vi "main 5th.vi"() -> ()   [LabVIEW 2013]
panel:
  out "From OD fit?":bool
  in  "Current file num":i32
  in  "Fitting Results Save Path":string[](array[string])
  in  "Initial guess values":dbl[](array[numeric])
  out "Latest image data":dbl[][](array[numeric])
  in  "Fitting Type":u16(ring)
  in  "Force Guess?":bool
  out "best fit parameters":dbl[](array[numeric])
  in  "Reset process index":bool
  out "ROI Height":u32
  out "ROI Width":u32
  out "OD image":dbl[][](graph)
  out "Process Index":i32
  out "External Trigger":bool
  out "XY图":cluster{i32[], dbl[]}[](graph)
  in  "OD fit":bool
  in  "OD num":i32
  out "Fit Done":bool
  in  "Exit":bool
  out "XY图 2":cluster{i32[], dbl[]}[](graph)
  in  "Auto Split":bool
  in  "Fit":bool
  in  "Open File":bool
  in  "Auto Fit":bool
  in  "Stop":bool
  in  "Aquire":bool
  in  "Fitting Config":bool
  in  "Camera Config":bool
  in  "Initialize":bool
  in  "Live Image Display":refnum<k7>(container)
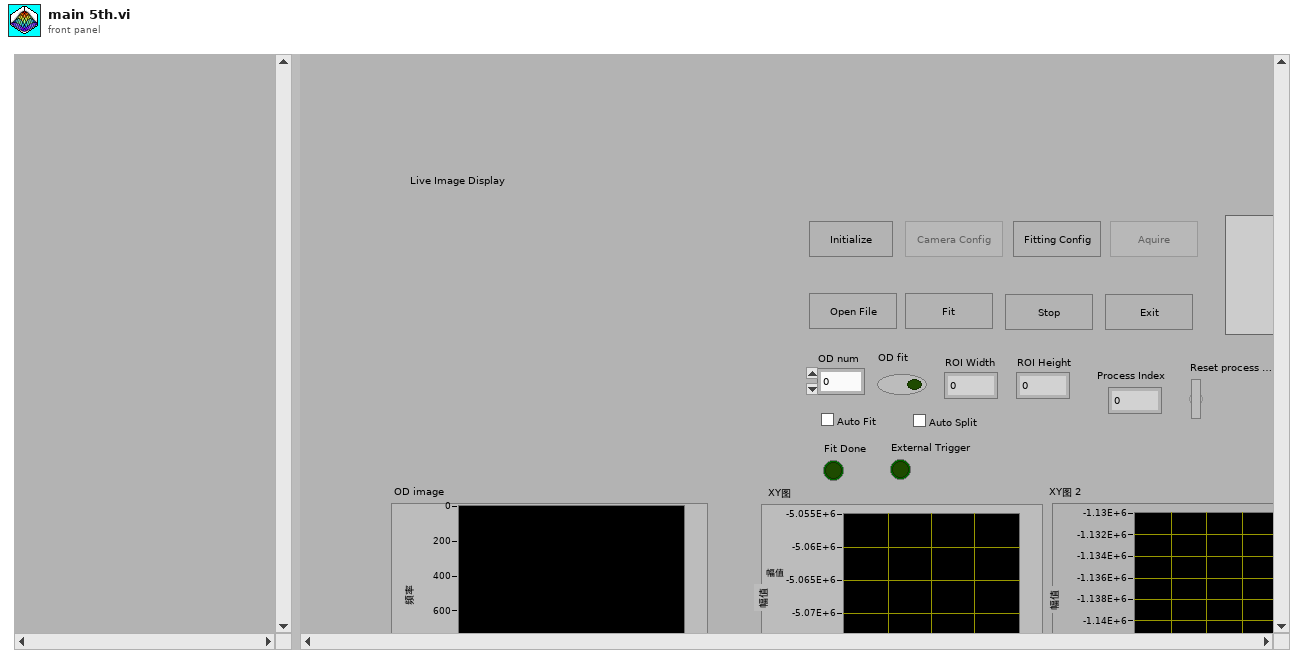
[diagram p1: front panel]
types:
  T1 = enum8{"Enabled", "Disabled", "Disabled and Grayed Out"}
  T2 = typedef "Image Type" = u32
  T3 = typedef "IMAQ Image.ctl" = refnum<image>
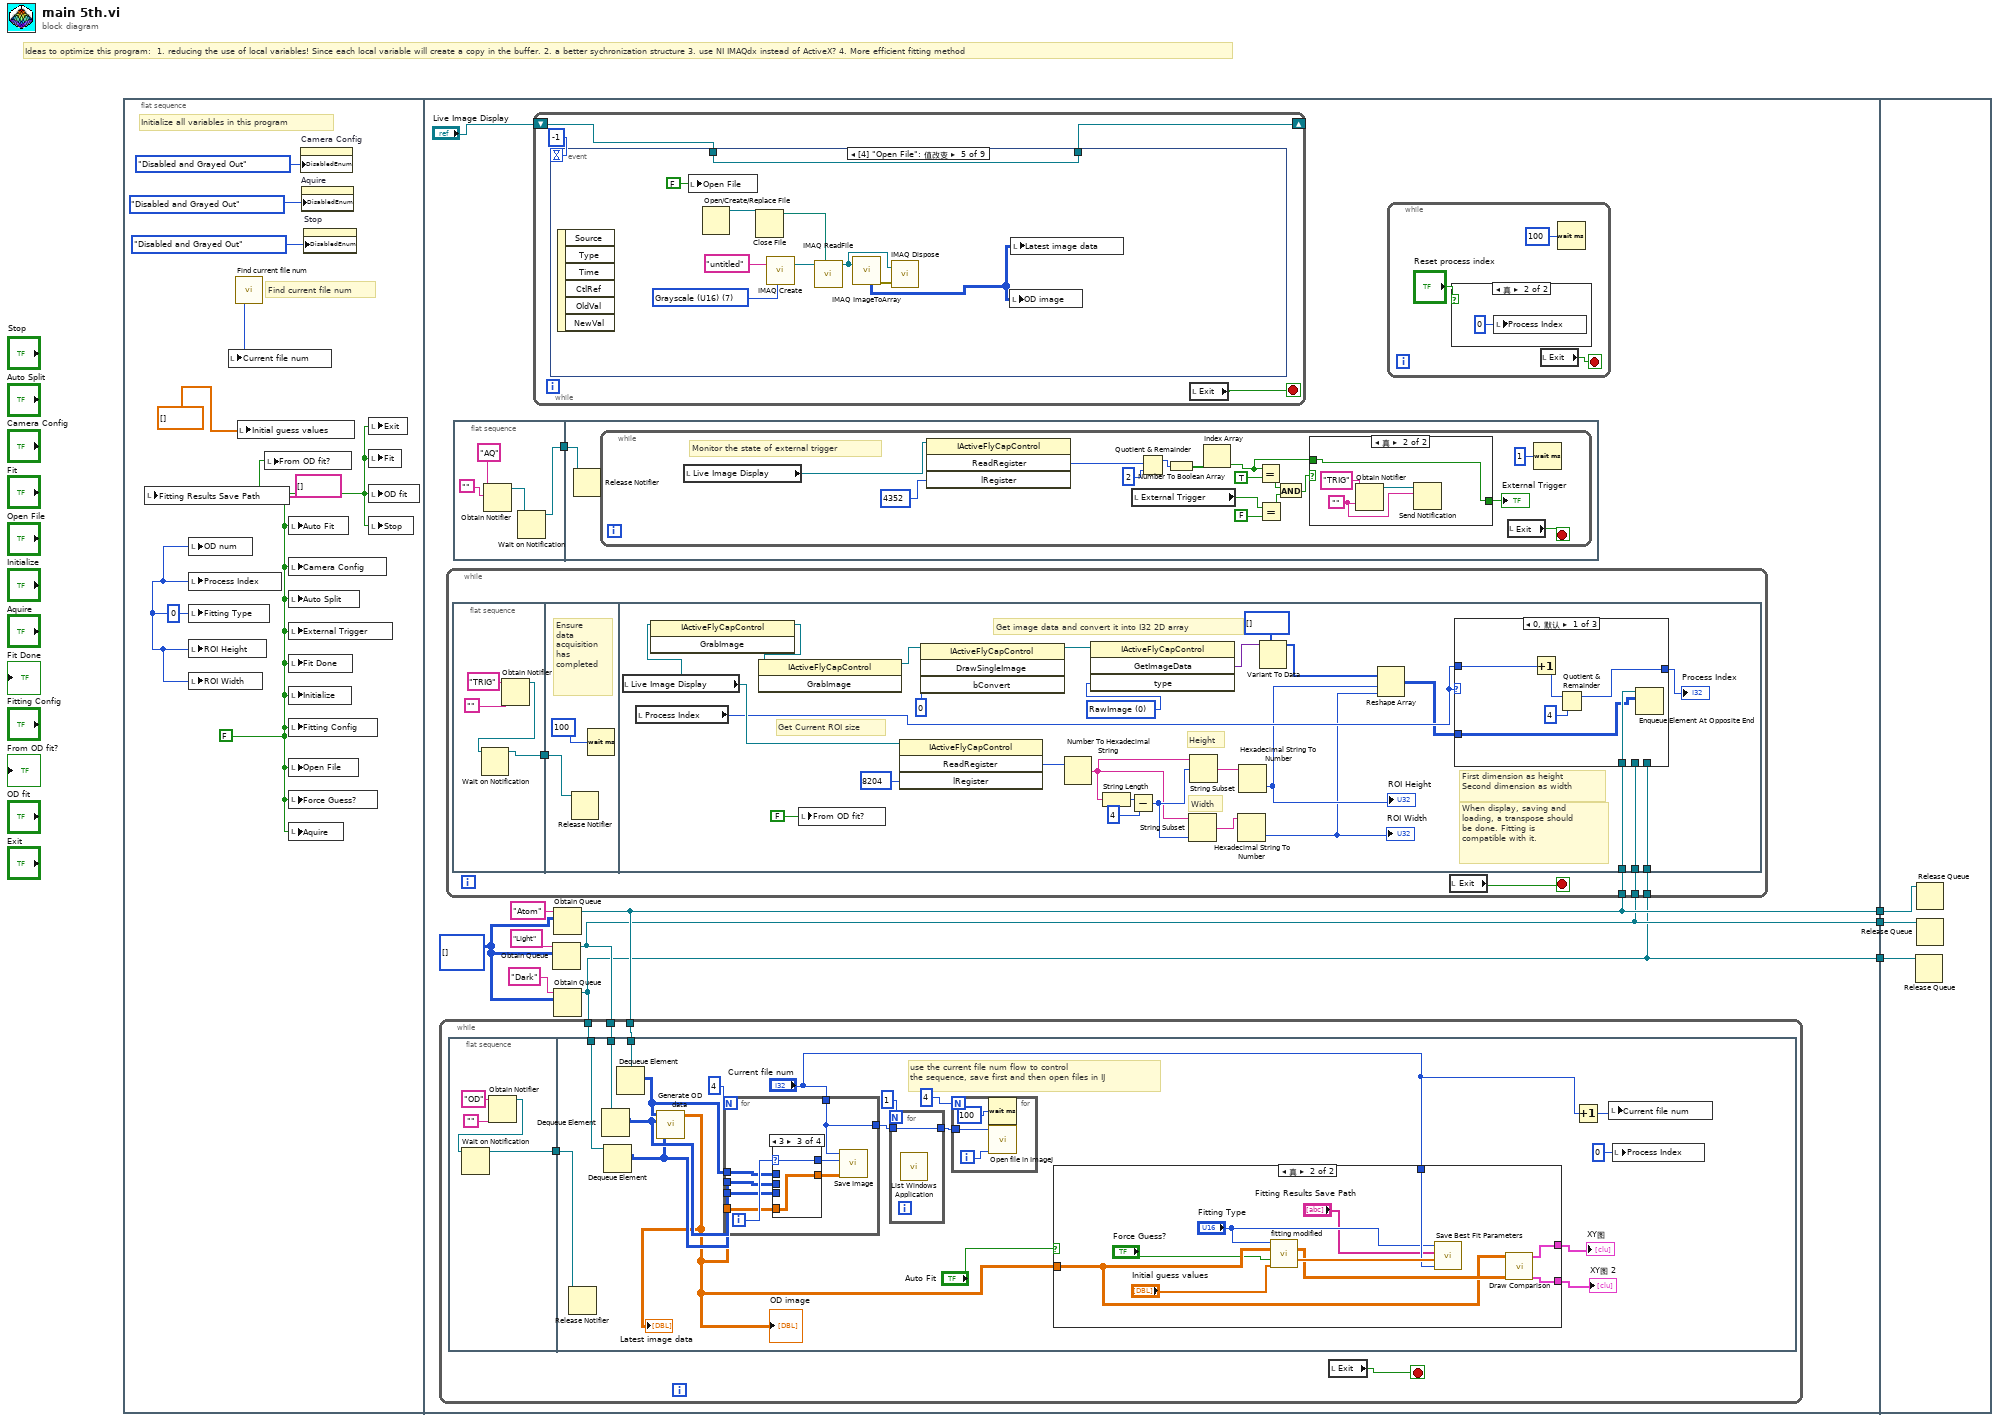
[diagram p0: block diagram]
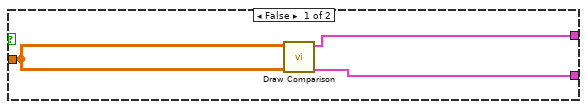
[diagram p3: hidden frame]
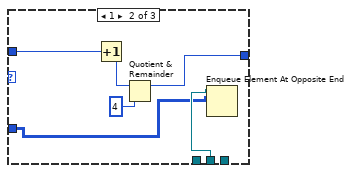
[diagram p8: hidden frame]
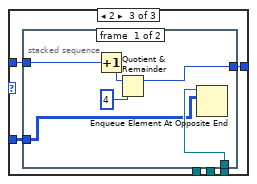
[diagram p9: hidden frame]
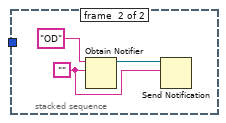
[diagram p10: hidden frame]
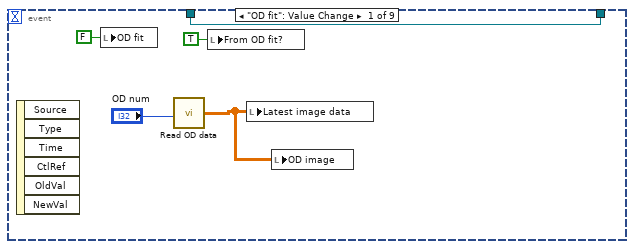
[diagram p11: hidden frame]
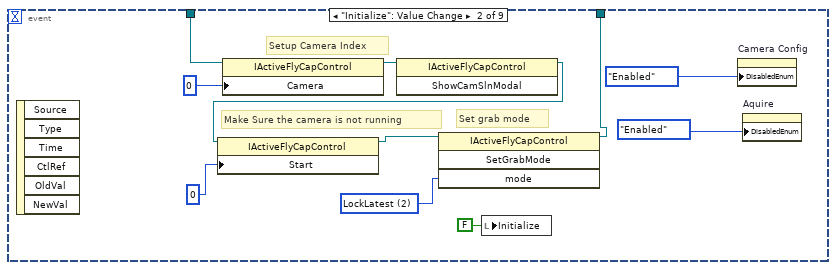
[diagram p12: hidden frame]
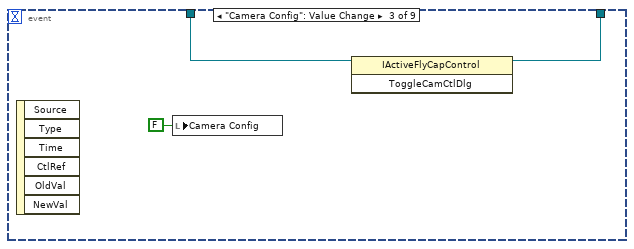
[diagram p13: hidden frame]
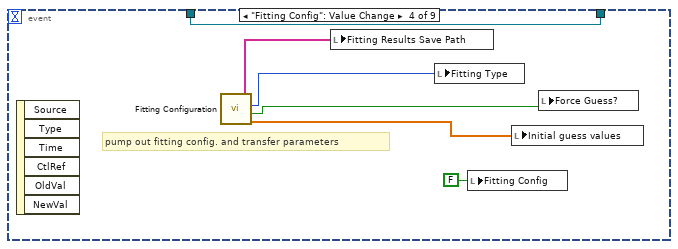
[diagram p14: hidden frame]
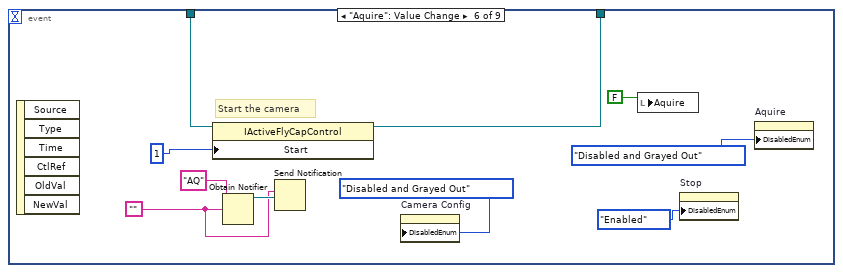
[diagram p15: hidden frame]
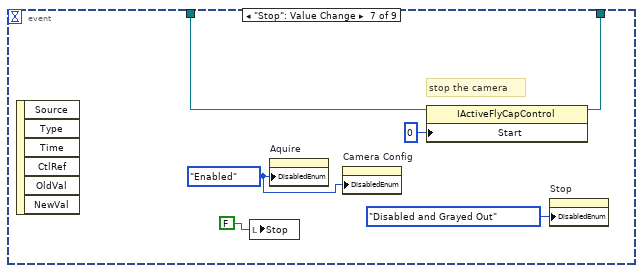
[diagram p16: hidden frame]
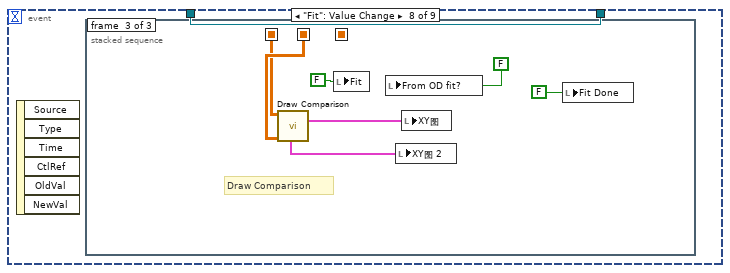
[diagram p17: hidden frame]
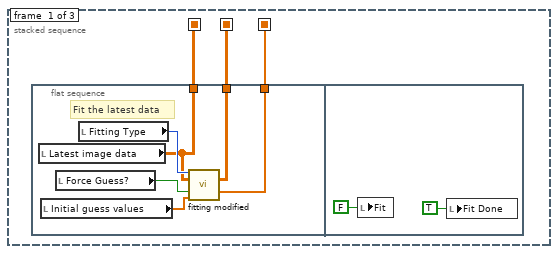
[diagram p18: hidden frame]
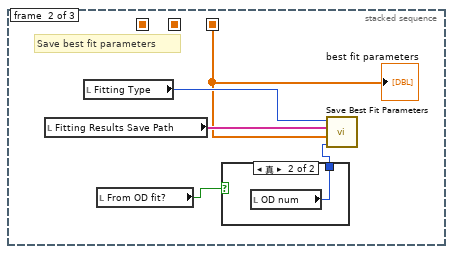
[diagram p19: hidden frame]
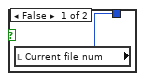
[diagram p20: hidden frame]
diagram:
  # "Ideas to optimize this program:  1. reducing the use of local variables! Since each local variable will create a copy in the buffer. 2. a better sychronization structure 3. use NI IMAQdx instead of ActiveX? 4. More efficient fitting method"
  n1 = flat-sequence {
    tunnel: [w15] -> w3
    tunnel: [w14] -> w2
    tunnel: [w13] -> w1
    tunnel: w3 -> [w258]
    tunnel: w2 -> [w257]
    tunnel: w1 -> [w256]
    frame #0 {
      w7 = 0 ("OD num")
      w5 = FALSE ("Aquire")
      # "Find current file num"
      # "Initialize all variables in this program"
      n2 = local write "Fitting Results Save Path"(string[] [] ("Fitting Results Save Path")) -> ()
      n3 = local write "OD num"(w7) -> ()
      n4 = local write "Process Index"(w7) -> ()
      n5 = local write "Fitting Type"(w7) -> ()
      n6 = local write "ROI Height"(w7) -> ()
      n7 = local write "ROI Width"(w7) -> ()
      n8 = call "Find current file num.vi"() -> ("Current File Num"=w4:u16)  [unwired: 2 in]
      n9 = local write "Current file num"(w4) -> ()
      n10 = local write "Initial guess values"(dbl[] [] ("Best fit parameters")) -> ()
      n11 = local write "From OD fit?"(w5) -> ()
      n12 = local write "Auto Fit"(w5) -> ()
      n13 = local write "Camera Config"(w5) -> ()
      n14 = local write "Auto Split"(w5) -> ()
      n15 = local write "External Trigger"(w5) -> ()
      n16 = local write "Fit Done"(w5) -> ()
      n17 = local write "Initialize"(w5) -> ()
      n18 = local write "Fitting Config"(w5) -> ()
      n19 = local write "Open File"(w5) -> ()
      n20 = local write "Force Guess?"(w5) -> ()
      n21 = local write "Aquire"(w5) -> ()
      n22 = property on="Camera Config" class="Bool (严格)"("DisabledEnum"=T1."Disabled and Grayed Out" ("禁用")) -> ()  [unwired: 2 in, 2 out]
      n23 = property on="Aquire" class="Bool (严格)"("DisabledEnum"=T1."Disabled and Grayed Out" ("禁用")) -> ()  [unwired: 2 in, 2 out]
      n24 = property on="Stop" class="Bool (严格)"("DisabledEnum"=T1."Disabled and Grayed Out" ("禁用")) -> ()  [unwired: 2 in, 2 out]
      n25 = local write "Exit"(w5) -> ()
      n26 = local write "Fit"(w5) -> ()
      n27 = local write "OD fit"(w5) -> ()
      n28 = local write "Stop"(w5) -> ()
    }
    frame #1 {
      w16 = i32[][] [] ("输出数组")
      n29 = flat-sequence {
        tunnel: [w86] -> w20
        tunnel: w20 -> [w90]
        frame #0 {
          n30 = Obtain Notifier(name (unnamed)="AQ" ("名称（未命名）"), notification data type="") -> (notifier out=w88:refnum<notifier>)  [unwired: 2 in, 2 out]
          n31 = Wait on Notification(notifier=w88) -> (notifier out=w86:refnum<notifier>)  [unwired: 3 in, 3 out]
        }
        frame #1 {
          n32 = Release Notifier(notifier=w90) -> ()  [unwired: 2 in, 3 out]
          n33 = while {
            stop <- w106 stop-if-true
            # "Monitor the state of external trigger"
            n34 = local read "Live Image Display"() -> (w105:refnum<k7>)
            n35 = invoke class="IActiveFlyCapControl" method="ReadRegister"(reference=w105, "lRegister"=u32 4352) -> ("ReadRegister"=w103:u32)  [unwired: 2 in, 3 out]
            n36 = local read "External Trigger"() -> (w98:bool)
            n37 = Quotient & Remainder(x=w103, y=u32 2) -> (x-y*floor(x/y)=w101:u32)  [unwired: 1 out]
            n38 = Number To Boolean Array(number=w101) -> (Boolean array=w100:bool[])
            n39 = Index Array(array=w100) -> (element=w93:bool)  [unwired: 1 in]
            n40 = Equal?(x=w93, y=TRUE) -> (x = y?=w95:bool)
            n41 = Equal?(x=w98, y=FALSE) -> (x = y?=w96:bool)
            n42 = And(x=w95, y=w96) -> (x .and. y?=w94:bool)
            n43 = case shown="真" w94 {
              tunnel: w93 -> [w107 w108]
              tunnel: [w107 w108] -> w91
              frame False {
              }
              frame True {
                w109 = ""
                n44 = Obtain Notifier(name (unnamed)="TRIG" ("名称（未命名）"), notification data type=w109) -> (notifier out=w110:refnum<notifier>)  [unwired: 2 in, 2 out]
                n45 = Send Notification(notification=w109, notifier=w110) -> ()  [unwired: 1 in, 2 out]
              }
            }
            "External Trigger" <- w91
            n46 = local read "Exit"() -> (w106:bool)
            n47 = Wait (ms)(milliseconds to wait=u32 1 ("等待时间（毫秒）")) -> ()  [unwired: 1 out]
          }
        }
      }
      n48 = while {
        shift-right: [w174] -> _
        shift-left: "Live Image Display" -> [w175]
        stop <- w177 stop-if-true
        n49 = event shown="[4] \"Open File\": 值改变" {
          selector: _ -> [_ _ _ _ _ _ _ _ _]
          dyn-events: _ -> [_ _ _ _ _ _ _ _ _]
          timeout: -1 -> [_ _ _ _ _ _ _ _ _]
          tunnel: w175 -> [w178 w187 w195 w197 w211 w214 w225 w229 w255]
          tunnel: [w178 w183 w194 w197 w211 w213 w224 w229 w255] -> w174
          event "OD fit": Value Change {
            n50 = event-data() -> ()  [unwired: 1 in, 6 out]
            n51 = local write "OD fit"(FALSE ("OD fit")) -> ()
            n52 = call "Read OD data.vi"("OD num"="OD num") -> ("OD data"=w180:dbl[][])  [unwired: 4 in]
            n53 = local write "From OD fit?"(TRUE ("From OD fit?")) -> ()
            n54 = local write "Latest image data"(w180) -> ()
            n55 = local write "OD image"(w180) -> ()
          }
          event "Initialize": Value Change {
            w191 = 2 items=["FreeRunning", "LockNext", "LockLatest"] ("mode")
            # "Setup Camera Index"
            # "Set grab mode"
            # "Make Sure the camera is not running"
            n56 = event-data() -> ()  [unwired: 1 in, 6 out]
            n57 = property class="IActiveFlyCapControl"(reference=w187, "Camera"=0 ("Start")) -> (reference out=w190:refnum<k7>)  [unwired: 1 in, 1 out]
            n58 = invoke class="IActiveFlyCapControl" method="ShowCamSlnModal"(reference=w190) -> (reference out=w186:refnum<k7>)  [unwired: 2 in, 2 out]
            n59 = property class="IActiveFlyCapControl"(reference=w186, "Start"=0 ("Camera")) -> (reference out=w185:refnum<k7>)  [unwired: 1 in, 1 out]
            n60 = invoke class="IActiveFlyCapControl" method="SetGrabMode"(reference=w185, "mode"=w191) -> (reference out=w183:refnum<k7>)  [unwired: 2 in, 3 out]
            n61 = local write "Initialize"(FALSE ("Initialize")) -> ()
            n62 = property on="Camera Config" class="Bool (严格)"("DisabledEnum"=T1."Enabled" ("禁用")) -> ()  [unwired: 2 in, 2 out]
            n63 = property on="Aquire" class="Bool (严格)"("DisabledEnum"=T1."Enabled" ("禁用")) -> ()  [unwired: 2 in, 2 out]
          }
          event "Camera Config": Value Change {
            n64 = event-data() -> ()  [unwired: 1 in, 6 out]
            n65 = local write "Camera Config"(FALSE ("Camera Config")) -> ()
            n66 = invoke class="IActiveFlyCapControl" method="ToggleCamCtlDlg"(reference=w195) -> (reference out=w194:refnum<k7>)  [unwired: 2 in, 2 out]
          }
          event "Fitting Config": Value Change {
            # "pump out fitting config. and transfer parameters"
            n67 = event-data() -> ()  [unwired: 1 in, 6 out]
            n68 = call "Fitting Configuration.vi"() -> ("intial guess"=w198:dbl[], "Force Guess？"=w199:bool, "Fitting Type"=w201:u16, "Fitting Results Save Path"=w200:string[])  [unwired: 5 in]
            n69 = local write "Fitting Results Save Path"(w200) -> ()
            n70 = local write "Fitting Type"(w201) -> ()
            n71 = local write "Fitting Config"(FALSE ("Fitting Config")) -> ()
            n72 = local write "Initial guess values"(w198) -> ()
            n73 = local write "Force Guess?"(w199) -> ()
          }
          event "Open File": Value Change {
            w210 = T2 7 items=["Grayscale (U8)", "Grayscale (I16)", "Grayscale (SGL)", "Complex (CSG)", "RGB (U32)", "HSL (U32)", "RGB (U64)", "Grayscale (U16)"] ("Image Type")
            n74 = event-data() -> ()  [unwired: 1 in, 6 out]
            n75 = local write "Open File"(FALSE ("Open File")) -> ()
            n76 = Open/Create/Replace File() -> (refnum out=w204:refnum<file>)  [unwired: 6 in, 2 out]
            n77 = Close File(refnum=w204) -> (path=w203:path)  [unwired: 1 in, 1 out]
            n78 = call "IMAQ Create"("Image Name"="untitled", "Image Type"=w210) -> ("New Image"=w209:T3)  [unwired: 3 in, 1 out]
            n79 = call "IMAQ ReadFile"("File Path"=w203, "Image"=w209) -> ("Image Out"=w208:T3)  [unwired: 5 in, 4 out]
            n80 = call "IMAQ ImageToArray"("Image"=w208) -> ("Image Pixels (U16)"=w205:u16[][], "error out"=w207:errorcluster)  [unwired: 3 in, 3 out]
            n81 = call "IMAQ Dispose"("Image"=w208, "error in (no error)"=w207) -> ()  [unwired: 4 in, 1 out]
            n82 = local write "OD image"(w205) -> ()
            n83 = local write "Latest image data"(w205) -> ()
          }
          event "Aquire": Value Change {
            w216 = ""
            # "Start the camera"
            n84 = event-data() -> ()  [unwired: 1 in, 6 out]
            n85 = property class="IActiveFlyCapControl"(reference=w214, "Start"=1) -> (reference out=w213:refnum<k7>)  [unwired: 1 in, 1 out]
            n86 = Obtain Notifier(name (unnamed)="AQ" ("名称（未命名）"), notification data type=w216) -> (notifier out=w217:refnum<notifier>)  [unwired: 2 in, 2 out]
            n87 = Send Notification(notification=w216, notifier=w217) -> ()  [unwired: 1 in, 2 out]
            n88 = property on="Camera Config" class="Bool (严格)"("DisabledEnum"=T1."Disabled and Grayed Out" ("禁用")) -> ()  [unwired: 2 in, 2 out]
            n89 = local write "Aquire"(FALSE ("Initialize")) -> ()
            n90 = property on="Stop" class="Bool (严格)"("DisabledEnum"=T1."Enabled" ("禁用")) -> ()  [unwired: 2 in, 2 out]
            n91 = property on="Aquire" class="Bool (严格)"("DisabledEnum"=T1."Disabled and Grayed Out" ("禁用")) -> ()  [unwired: 2 in, 2 out]
          }
          event "Stop": Value Change {
            w223 = T1."Enabled" ("禁用")
            # "stop the camera"
            n92 = event-data() -> ()  [unwired: 1 in, 6 out]
            n93 = local write "Stop"(FALSE ("Initialize")) -> ()
            n94 = property on="Aquire" class="Bool (严格)"("DisabledEnum"=w223) -> ()  [unwired: 2 in, 2 out]
            n95 = property on="Camera Config" class="Bool (严格)"("DisabledEnum"=w223) -> ()  [unwired: 2 in, 2 out]
            n96 = property class="IActiveFlyCapControl"(reference=w225, "Start"=0) -> (reference out=w224:refnum<k7>)  [unwired: 1 in, 1 out]
            n97 = property on="Stop" class="Bool (严格)"("DisabledEnum"=T1."Disabled and Grayed Out" ("禁用")) -> ()  [unwired: 2 in, 2 out]
          }
          event "Fit": Value Change {
            n98 = event-data() -> ()  [unwired: 1 in, 6 out]
            n99 = stacked-sequence {
              seq-local: [w231 _ _] -> [_ _ w251]
              seq-local: [w232 _ _] -> [_ _ w249]
              seq-local: [w230 _ _] -> [_ w241 _]
              frame #0 {
                n100 = flat-sequence {
                  tunnel: [w235] -> w232
                  tunnel: [w234] -> w231
                  tunnel: [w233] -> w230
                  frame #0 {
                    # "Fit the latest data"
                    n101 = local read "Latest image data"() -> (w235:dbl[][])
                    n102 = local read "Initial guess values"() -> (w237:dbl[])
                    n103 = local read "Force Guess?"() -> (w238:bool)
                    n104 = local read "Fitting Type"() -> (w236:u16)
                    n105 = call "fitting modified.vi"("fitting type"=w236, "2D data"=w235, "force guess?"=w238, "intial guess value"=w237) -> ("best fit"=w234:dbl[][], "best fit parameters"=w233:dbl[])  [unwired: 9 in, 1 out]
                  }
                  frame #1 {
                    n106 = local write "Fit"(FALSE ("Fit")) -> ()
                    n107 = local write "Fit Done"(TRUE ("Fit Done")) -> ()
                  }
                }
              }
              frame #1 {
                # "Save best fit parameters"
                n108 = local read "Fitting Results Save Path"() -> (w244:string[])
                n109 = local read "Fitting Type"() -> (w245:u16)
                n110 = local read "From OD fit?"() -> (w243:bool)
                n111 = case shown="真" w243 {
                  tunnel: [w246 w247] -> w242
                  frame False {
                    n112 = local read "Current file num"() -> (w246:i32)
                  }
                  frame True {
                    n113 = local read "OD num"() -> (w247:i32)
                  }
                }
                n114 = call "Save Best Fit Parameters.vi"("Current File Num"=w242, "Best Fit Parameters"=w241, "Fitting Results Save Path"=w244, "Fitting Type"=w245) -> ()  [unwired: 8 in]
                "best fit parameters" <- w241
              }
              frame #2 {
                # "Draw Comparison"
                n115 = call "Draw Comparison.vi"("Best Fit"=w251, "Raw Data"=w249) -> ("Vertical Comparison"=w253:cluster{i32[], dbl[]}[], "Horizontal Comparison"=w254:cluster{i32[], dbl[]}[])  [unwired: 7 in]
                n116 = local write "Fit"(FALSE ("Initialize")) -> ()
                n117 = local write "From OD fit?"(FALSE ("From OD fit?")) -> ()
                n118 = local write "XY图 2"(w253) -> ()
                n119 = local write "XY图"(w254) -> ()
                n120 = local write "Fit Done"(FALSE ("Fit Done")) -> ()
              }
            }
          }
          event Timeout {
            n121 = event-data() -> ()  [unwired: 1 in, 3 out]
          }
        }
        n122 = local read "Exit"() -> (w177:bool)
      }
      n123 = Obtain Queue(name (unnamed)="Light" ("名称（未命名）"), element data type=w16) -> (queue out=w14:refnum<queue>)  [unwired: 3 in, 2 out]
      n124 = Obtain Queue(name (unnamed)="Atom" ("名称（未命名）"), element data type=w16) -> (queue out=w15:refnum<queue>)  [unwired: 3 in, 2 out]
      n125 = Obtain Queue(name (unnamed)="Dark" ("名称（未命名）"), element data type=w16) -> (queue out=w13:refnum<queue>)  [unwired: 3 in, 2 out]
      n126 = while {
        tunnel: w15 -> [w27]
        tunnel: w14 -> [w26]
        tunnel: w13 -> [w25]
        stop <- w29 stop-if-true
        n127 = flat-sequence {
          tunnel: [w30] -> w28
          tunnel: w28 -> [w52]
          tunnel: w27 -> [w50]
          tunnel: w26 -> [w48]
          tunnel: w25 -> [w46]
          frame #0 {
            n128 = Obtain Notifier(name (unnamed)="OD" ("名称（未命名）"), notification data type="") -> (notifier out=w31:refnum<notifier>)  [unwired: 2 in, 2 out]
            n129 = Wait on Notification(notifier=w31) -> (notifier out=w30:refnum<notifier>)  [unwired: 3 in, 3 out]
          }
          frame #1 {
            # "use the current file num flow to control \nthe sequence, save first and then open files in IJ"
            n130 = Release Notifier(notifier=w52) -> ()  [unwired: 2 in, 3 out]
            n131 = Dequeue Element(queue=w48) -> (element=w47:i32[][])  [unwired: 2 in, 3 out]
            n132 = Dequeue Element(queue=w46) -> (element=w45:i32[][])  [unwired: 2 in, 3 out]
            n133 = Dequeue Element(queue=w50) -> (element=w49:i32[][])  [unwired: 2 in, 3 out]
            n134 = call "Generate OD data.vi"("dark"=w45, "light"=w47, "atom"=w49) -> ("OD image"=w41:dbl[][])  [unwired: 3 in]
            "OD image" <- w41
            "Latest image data" <- w41
            n135 = for {
              N: 4 -> [_]
              tunnel: w49 -> [w76]
              tunnel: w47 -> [w75]
              tunnel: w45 -> [w74]
              tunnel: w41 -> [w73]
              tunnel: "Current file num" -> [w70]
              tunnel: [w70] -> w34
              i -> [w77]
              n136 = case shown="3" w77 {
                selector: w77 -> [w79 w81 w83 w85]
                tunnel: w76 -> [w78 _ _ _]
                tunnel: w75 -> [_ _ _ w84]
                tunnel: w74 -> [_ w80 _ _]
                tunnel: w73 -> [_ _ w82 _]
                tunnel: [w79 w81 w83 w85] -> w72
                tunnel: [w78 w80 w82 w84] -> w71
                frame 0, Default {
                }
                frame 2 {
                }
                frame 3 {
                }
                frame 1 {
                }
              }
              n137 = call "Save Image.vi"("Data"=w71, "Process Index"=w72, "Current File Num"=w70) -> ()  [unwired: 9 in]
            }
            n138 = for {
              N: 1 -> [_]
              tunnel: w34 -> [w53]
              tunnel: [w53] -> w36
              n139 = call "List Windows Application.vi"() -> ()  [unwired: 1 in]
            }
            n140 = for {
              N: 4 -> [_]
              tunnel: w36 -> [w56]
              i -> [w55]
              n141 = Wait (ms)(milliseconds to wait=u32 100) -> ()  [unwired: 1 out]
              n142 = call "Open file in ImageJ.vi"("Process Index"=w55, "Current File Num"=w56) -> ()  [unwired: 10 in]
            }
            n143 = case shown="真" "Auto Fit" {
              tunnel: w41 -> [w59 w66]
              tunnel: "Current file num" -> [_ w68]
              tunnel: [w58 w65] -> w42
              tunnel: [w57 w64] -> w43
              frame False {
                n144 = call "Draw Comparison.vi"("Best Fit"=w59, "Raw Data"=w59) -> ("Vertical Comparison"=w57:cluster{i32[], dbl[]}[], "Horizontal Comparison"=w58:cluster{i32[], dbl[]}[])  [unwired: 7 in]
              }
              frame True {
                n145 = call "fitting modified.vi"("fitting type"="Fitting Type", "2D data"=w66, "force guess?"="Force Guess?", "intial guess value"="Initial guess values") -> ("best fit"=w67:dbl[][], "best fit parameters"=w69:dbl[])  [unwired: 9 in, 1 out]
                n146 = call "Save Best Fit Parameters.vi"("Current File Num"=w68, "Best Fit Parameters"=w69, "Fitting Results Save Path"="Fitting Results Save Path", "Fitting Type"="Fitting Type") -> ()  [unwired: 8 in]
                n147 = call "Draw Comparison.vi"("Best Fit"=w67, "Raw Data"=w66) -> ("Vertical Comparison"=w64:cluster{i32[], dbl[]}[], "Horizontal Comparison"=w65:cluster{i32[], dbl[]}[])  [unwired: 7 in]
              }
            }
            "XY图" <- w42
            "XY图 2" <- w43
            n148 = Increment(x="Current file num") -> (x+1=w40:i32)
            n149 = local write "Current file num"(w40) -> ()
            n150 = local write "Process Index"(0 ("Process Index")) -> ()
          }
        }
        n151 = local read "Exit"() -> (w29:bool)
      }
      n152 = while {
        tunnel: w15 -> [w114]
        tunnel: w14 -> [w113]
        tunnel: w13 -> [w112]
        stop <- w116 stop-if-true
        n153 = flat-sequence {
          tunnel: [w117] -> w115
          tunnel: w115 -> [w122]
          tunnel: w114 -> [w128]
          tunnel: w113 -> [w127]
          tunnel: w112 -> [w126]
          frame #0 {
            n154 = Obtain Notifier(name (unnamed)="TRIG" ("名称（未命名）"), notification data type="") -> (notifier out=w118:refnum<notifier>)  [unwired: 2 in, 2 out]
            n155 = Wait on Notification(notifier=w118) -> (notifier out=w117:refnum<notifier>)  [unwired: 3 in, 3 out]
          }
          frame #1 {
            # "Ensure\ndata\nacquisition\nhas \ncompleted"
            n156 = Release Notifier(notifier=w122) -> ()  [unwired: 2 in, 3 out]
            n157 = Wait (ms)(milliseconds to wait=u32 100 ("等待时间（毫秒）")) -> ()  [unwired: 1 out]
          }
          frame #2 {
            w148 = 0 items=["RawImage", "ColorProcessedImage"] ("type")
            # "Get image data and convert it into I32 2D array"
            # "When display, saving and \nloading, a transpose should\nbe done. Fitting is \ncompatible with it."
            # "First dimension as height\nSecond dimension as width"
            # "Width"
            # "Height"
            # "Get Current ROI size"
            n158 = local read "Live Image Display"() -> (w135:refnum<k7>)
            n159 = local read "Process Index"() -> (w132:i32)
            n160 = invoke class="IActiveFlyCapControl" method="GrabImage"(reference=w135) -> (reference out=w124:refnum<k7>)  [unwired: 2 in, 2 out]
            n161 = invoke class="IActiveFlyCapControl" method="GrabImage"(reference=w124) -> (reference out=w123:refnum<k7>)  [unwired: 2 in, 2 out]
            n162 = local write "From OD fit?"(FALSE ("From OD fit?")) -> ()
            n163 = invoke class="IActiveFlyCapControl" method="ReadRegister"(reference=w135, "lRegister"=u32 8204) -> ("ReadRegister"=w145:u32)  [unwired: 2 in, 3 out]
            n164 = invoke class="IActiveFlyCapControl" method="DrawSingleImage"(reference=w123, "bConvert"=0) -> (reference out=w134:refnum<k7>)  [unwired: 2 in, 3 out]
            n165 = Number To Hexadecimal String(2:w145) -> (0:w141:string)  [unwired: 1 in]
            n166 = invoke class="IActiveFlyCapControl" method="GetImageData"(reference=w134, "type"=w148) -> ("GetImageData"=w146:variant)  [unwired: 2 in, 3 out]
            n167 = String Length(string=w141) -> (length=w144:i32)
            n168 = Subtract(x=w144, y=4) -> (x-y=w142:i32)
            n169 = String Subset(string=w141, length (rest)=w142) -> (substring=w138:string)  [unwired: 1 in]
            n170 = String Subset(string=w141, offset (0)=w142) -> (substring=w139:string)  [unwired: 1 in]
            n171 = Hexadecimal String To Number(string=w138) -> (number=w129:u32)  [unwired: 2 in, 1 out]
            "ROI Width" <- w129
            n172 = Hexadecimal String To Number(string=w139) -> (number=w130:u32)  [unwired: 2 in, 1 out]
            "ROI Height" <- w130
            n173 = Variant To Data(type=i32[] [], Variant=w146) -> (data=w137:i32[])  [unwired: 1 in, 1 out]
            n174 = Reshape Array(w137, w130, w129) -> (w131:i32[][])
            n175 = case shown="0, 默认" w132 {
              tunnel: w132 -> [w152 w158 w164]
              tunnel: w131 -> [w149 w155 w163]
              tunnel: w128 -> [w150 _ _]
              tunnel: w127 -> [_ w156 _]
              tunnel: w126 -> [_ _ w162]
              tunnel: [w151 w157 w161] -> w125
              frame 0, Default {
                n176 = Increment(x=w152) -> (x+1=w153:i32)
                n177 = Quotient & Remainder(x=w153, y=4) -> (x-y*floor(x/y)=w151:i32)  [unwired: 1 out]
                n178 = Enqueue Element At Opposite End(queue=w150, element=w149) -> ()  [unwired: 2 in, 3 out]
              }
              frame 1 {
                n179 = Increment(x=w158) -> (x+1=w159:i32)
                n180 = Quotient & Remainder(x=w159, y=4) -> (x-y*floor(x/y)=w157:i32)  [unwired: 1 out]
                n181 = Enqueue Element At Opposite End(queue=w156, element=w155) -> ()  [unwired: 2 in, 3 out]
              }
              frame 2 {
                n182 = stacked-sequence {
                  tunnel: w164 -> [w168 _]
                  tunnel: w163 -> [w165 _]
                  tunnel: w162 -> [w166 _]
                  tunnel: [w167 _] -> w161
                  frame #0 {
                    n183 = Increment(x=w168) -> (x+1=w169:i32)
                    n184 = Quotient & Remainder(x=w169, y=4) -> (x-y*floor(x/y)=w167:i32)  [unwired: 1 out]
                    n185 = Enqueue Element At Opposite End(queue=w166, element=w165) -> ()  [unwired: 2 in, 3 out]
                  }
                  frame #1 {
                    w171 = ""
                    n186 = Obtain Notifier(name (unnamed)="OD" ("名称（未命名）"), notification data type=w171) -> (notifier out=w173:refnum<notifier>)  [unwired: 2 in, 2 out]
                    n187 = Send Notification(notification=w171, notifier=w173) -> ()  [unwired: 1 in, 2 out]
                  }
                }
              }
            }
            "Process Index" <- w125
          }
        }
        n188 = local read "Exit"() -> (w116:bool)
      }
      n189 = while {
        stop <- w23 stop-if-true
        n190 = case shown="真" "Reset process index" {
          frame False {
          }
          frame True {
            n191 = local write "Process Index"(0 ("Process Index")) -> ()
          }
        }
        n192 = local read "Exit"() -> (w23:bool)
        n193 = Wait (ms)(milliseconds to wait=u32 100 ("等待时间（毫秒）")) -> ()  [unwired: 1 out]
      }
    }
    frame #2 {
      n194 = Release Queue(queue=w256) -> ()  [unwired: 2 in, 3 out]
      n195 = Release Queue(queue=w258) -> ()  [unwired: 2 in, 3 out]
      n196 = Release Queue(queue=w257) -> ()  [unwired: 2 in, 3 out]
    }
  }
